vi "check for portrait.vi"(8 "error in (no error)":errorcluster, 11 "path":path) -> (0 "error out":errorcluster, 1 "imageHeight":i32, 2 "imageWidth":i32, 3 "Boolean":bool)   [LabVIEW 2023]
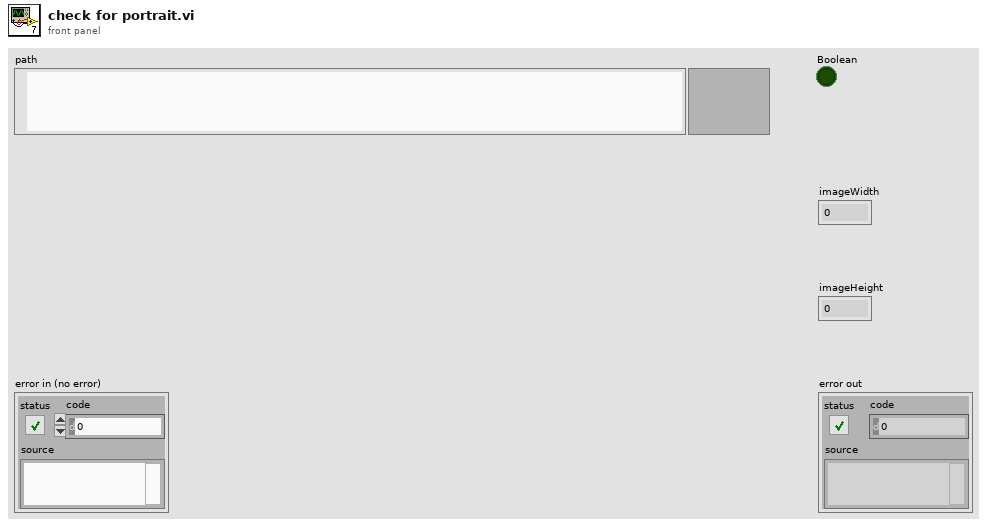
[diagram p1: front panel]
types:
  T1 = enum16{"271 - Make", "272 - Model", "274 - Orientation", "36867 - Date Orginal", "36868 - Date Digitize", "40962 - Width", "40963 - Height"}[]
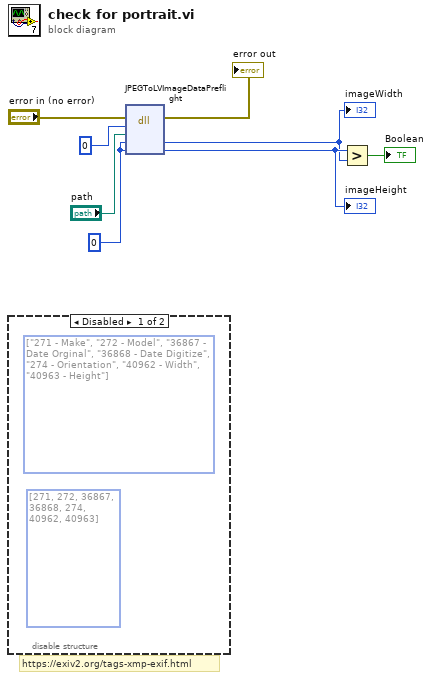
[diagram p0: block diagram]
diagram:
  w8 = 0
  # "https://exiv2.org/tags-xmp-exif.html"
  n1 = disable-structure shown="Disabled" {
    frame Disabled {
      (unwired) T1 [enum."271 - Make", enum."272 - Model", enum."36867 - Date Orginal", enum."36868 - Date Digitize", enum."274 - Orientation", enum."40962 - Width", enum."40963 - Height"] items=["271 - Make", "272 - Model", "274 - Orientation", "36867 - Date Orginal", "36868 - Date Digitize", "40962 - Width", "40963 - Height"]
      (unwired) i32[] [271, 272, 36867, 36868, 274, 40962, 40963]
    }
    frame Enabled {
    }
  }
  n2 = dll-call lib="LabVIEW" fn="JPEGToLVImageDataPreflight"(error in="error in (no error)", "return type"=0, "filename"="path", "imageWidth"=w8, "imageHeight"=w8) -> (error out=→"error out":errorcluster, "imageWidth"=w2:i32, "imageHeight"=w4:i32)  [unwired: 3 in, 1 out]
  "imageWidth" <- w2
  "imageHeight" <- w4
  n3 = Greater?(x=w4, y=w2) -> (0:→"Boolean":bool)
